vi "Quantizer.vi"   [LabVIEW 2017, in "NI_AdvCtrl_nonlinear.lvlib"]
doc: "LabVIEW no longer supports this VI. You can obtain similar functionality by installing the LabVIEW Simulation Module.\n\nQuantizes an input signal. It is output=[input/quantization interval]*quantization interval."
uses:
  <vilib>/addons/control/advanced/NI_AdvCtrl_nonlinear.lvlib
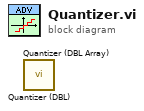
[diagram p0: block diagram]
diagram:
  n1 = call <vilib>:"Quantizer (DBL).vi"() -> ()  [unwired: 3 in, 1 out]
  n2 = call <vilib>:"Quantizer (DBL Array).vi"() -> ()  [unwired: 3 in, 1 out]
